vi "time.vi"(4 "Låst BPM":i32, 5 "project-param in":T3, 6 "Lås BPM":bool, 7 "Time Signatures":T1, 9 "Lower BPM":i32, 10 "Upper BPM":i32, 11 "Song structure":T2 {"Outro %" format="%#_13g"; "Solo %" format="%#_13g"; "Bridge %" format="%#_13g"; "Intro %" format="%#_13g"}) -> (3 "project-param out":T3)   [LabVIEW 2019]
uses:
  Project Parameters.ctl
  song-structure.ctl
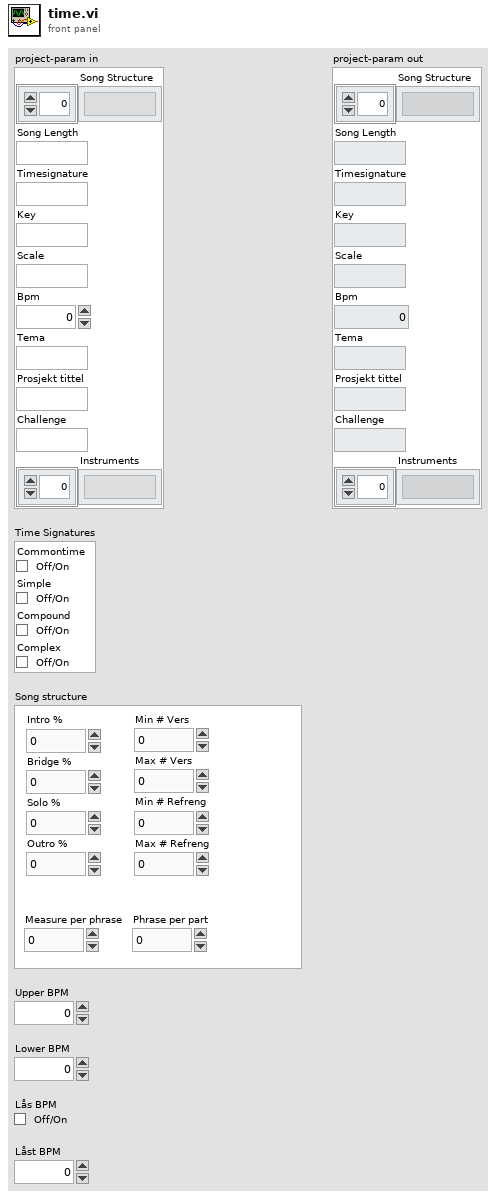
[diagram p1: front panel]
types:
  T1 = cluster{"Commontime":bool, "Simple":bool, "Compound":bool, "Complex":bool}
  T2 = typedef "song-structure.ctl" = cluster{"Intro %":dbl, "Bridge %":dbl, "Solo %":dbl, "Outro %":dbl, "Min # Vers":i32, "Max # Vers":i32, "Min # Refreng":i32, "Max # Refreng":i32, "Measure per phrase":i32, "Phrase per part":i32}
  T3 = typedef "Project Parameters.ctl" = cluster{"Song Structure":string[], "Song Length":string, "Timesignature":string, "Key":string, "Scale":string, "Bpm":i32, "Tema":string, "Prosjekt tittel":string, "Challenge":string, "Instruments":string[]}
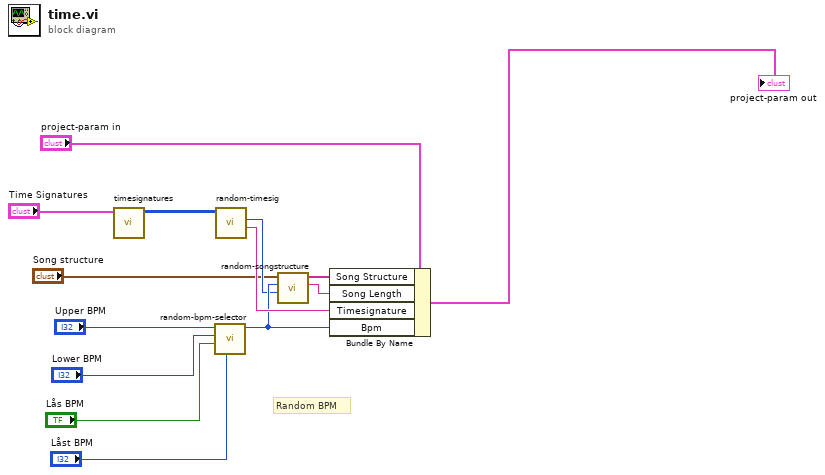
[diagram p0: block diagram]
diagram:
  # "Random BPM"
  n1 = call "timesignatures.vi"("Time Signatures"="Time Signatures") -> ("appended array"=w6:i32[][])  [unwired: 10 in]
  n2 = call "random-bpm-selector.vi"("Låst BPM in"="Låst BPM", "Lås BPM"="Lås BPM", "Lower BPM"="Lower BPM", "Upper BPM"="Upper BPM") -> ("BPM out"=w10:i32)  [unwired: 7 in]
  n3 = call "random-timesig.vi"("appended array"=w6) -> ("String"=w11:string, "Numeric"=w8:i32)  [unwired: 8 in, 1 out]
  n4 = call "random-songstructure.vi"("Numeric"=w8, "Låst BPM in"=w10, "Song structure"="Song structure") -> ("String"=w12:string, "Song Structure"=w13:string[])  [unwired: 7 in]
  n5 = Bundle By Name(cluster="project-param in", "Song Structure"=w13, "Song Length"=w12, "Timesignature"=w11, "Bpm"=w10) -> (→"project-param out":T3)
